vi "Test CML UI API.vi"() -> ()   [LabVIEW 2020]
doc: "CML UI API Tester.\n_____\nBased on DQMH Project Template 7.0.1.1316."
uses:
  <vilib>/Utility/error.llb/DialogType.ctl
  CML UI.lvlib
  <vilib>/Peloton/Peloton Config/DCFG Framework/Peloton_lib_DCFG Framework.lvlib
panel:
  in  "Views":string(combo)
  in  "Show DCFG Framework":bool
  in  "Show Diagram on Init":bool
  out "last error":errorcluster
  in  "Show Block Diagram":bool
  in  "Stop Module":bool
  in  "Start Module":bool
  in  "Hide Module Panel":bool
  in  "Show Module Panel":bool
  out "Status":string
  out "Module Running?":bool
  # "This VI tests the API for the Module."
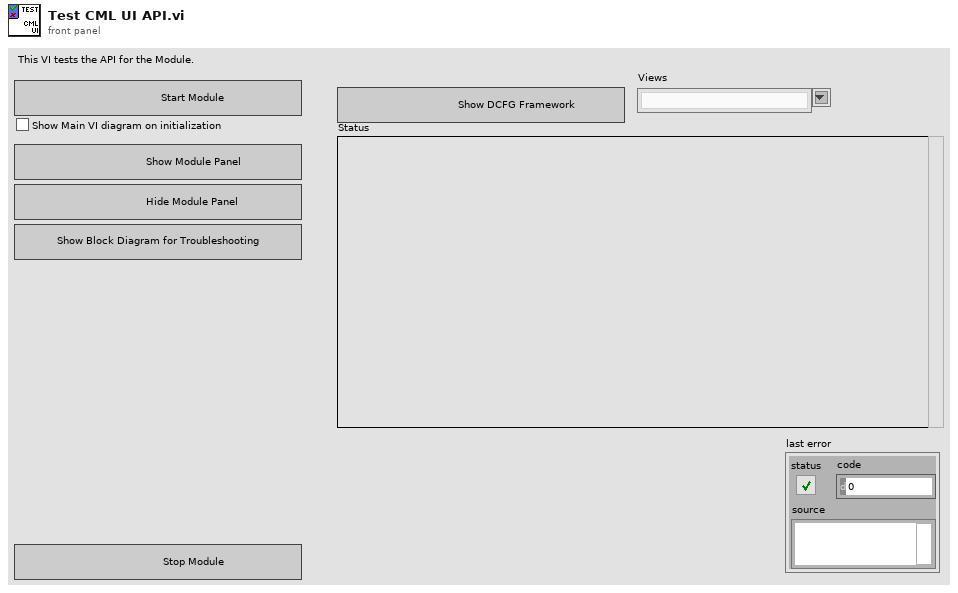
[diagram p1: front panel]
types:
  T1 = typedef "CML UI.lvlib/Broadcast Events--cluster.ctl" = cluster{"Module Did Init":refnum<user-event>, "Status Updated":refnum<user-event>, "Error Reported":refnum<user-event>, "Module Did Stop":refnum<user-event>, "Update Module Execution Status":refnum<user-event>}
  T2 = typedef "Peloton_lib_DCFG Framework.lvlib/Broadcast Events--cluster.ctl" = cluster{"Module Did Init":refnum<user-event>, "Status Updated":refnum<user-event>, "Error Reported":refnum<user-event>, "Module Did Stop":refnum<user-event>, "Update Module Execution Status":refnum<user-event>, "View Changed":refnum<user-event>, "Main Window Closed":refnum<user-event>, "Configuration Committed":refnum<user-event>, "Configuration Canceled":refnum<user-event>, "Views List Updated":refnum<user-event>, "Config Folder Path Updated":refnum<user-event>}
  T3 = typedef "DialogType.ctl" = u16
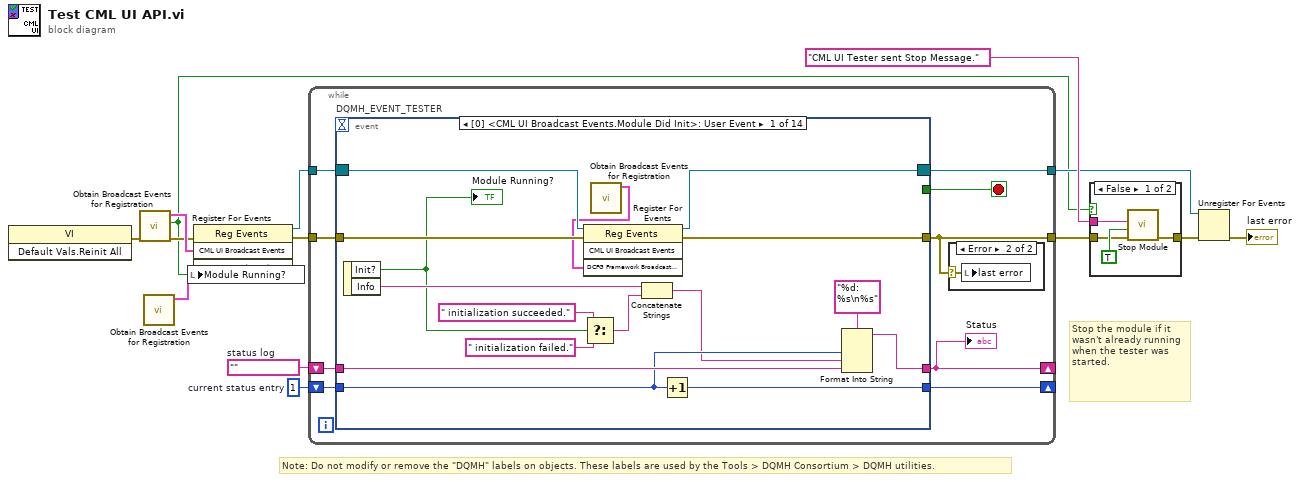
[diagram p0: block diagram]
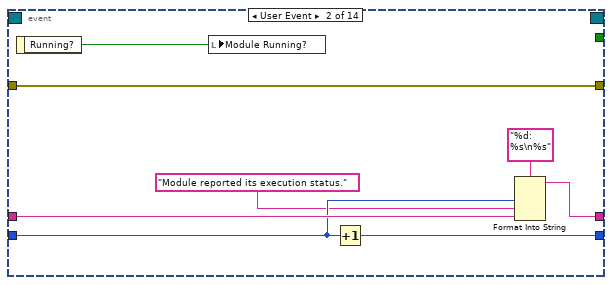
[diagram p3: hidden frame]
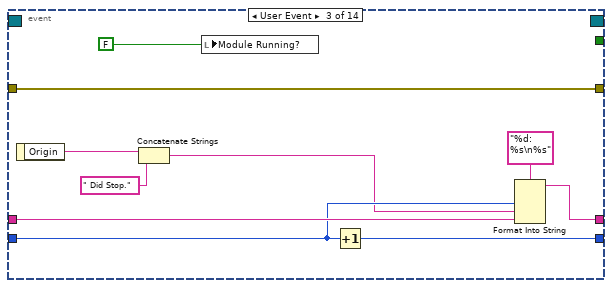
[diagram p4: hidden frame]
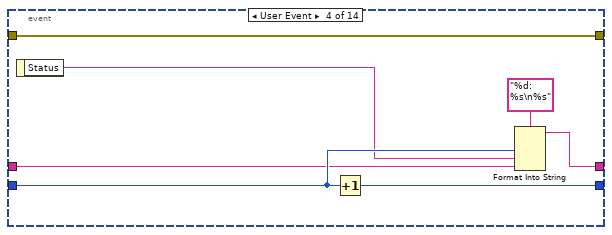
[diagram p5: hidden frame]
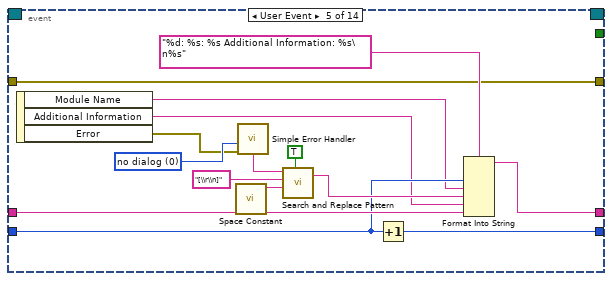
[diagram p6: hidden frame]
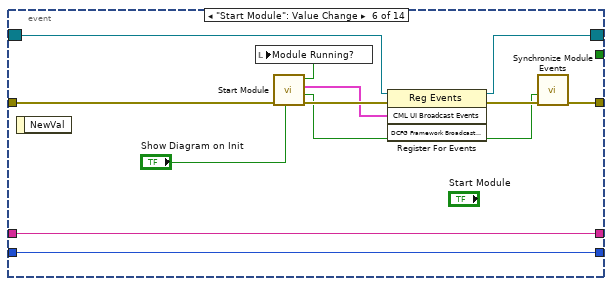
[diagram p7: hidden frame]
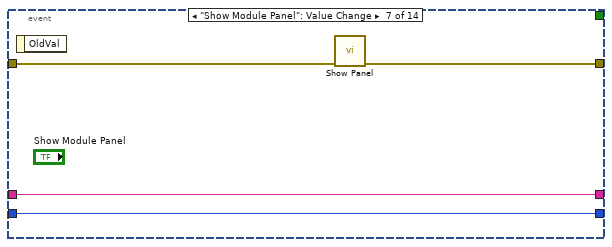
[diagram p8: hidden frame]
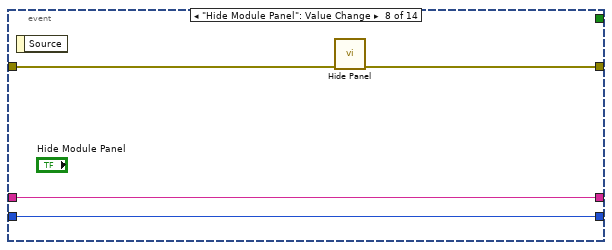
[diagram p9: hidden frame]
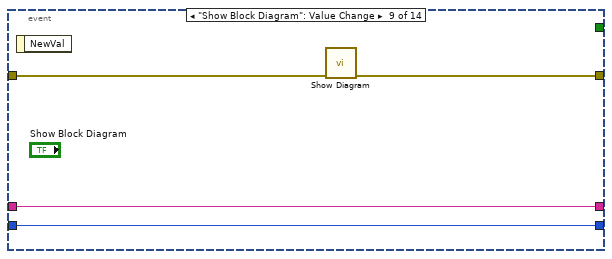
[diagram p10: hidden frame]
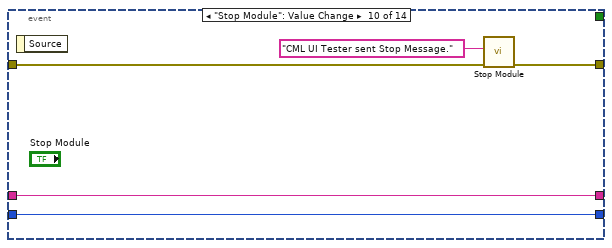
[diagram p11: hidden frame]
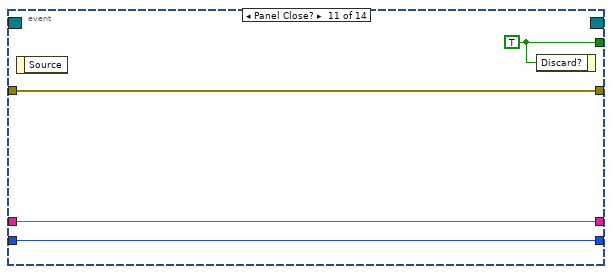
[diagram p12: hidden frame]
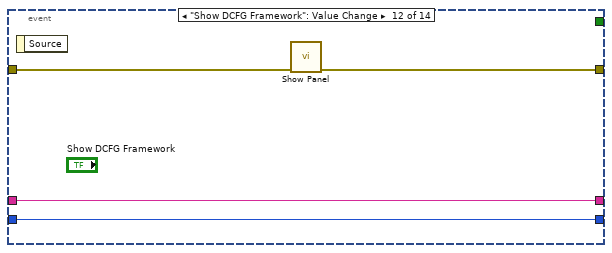
[diagram p13: hidden frame]
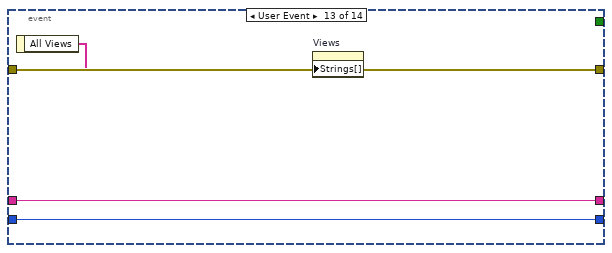
[diagram p14: hidden frame]
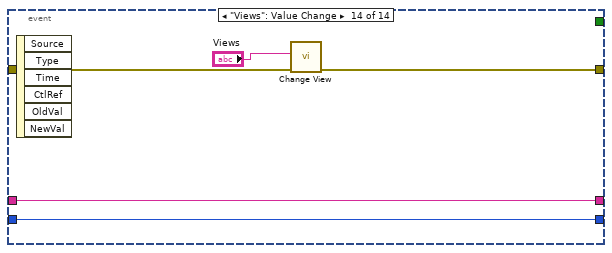
[diagram p15: hidden frame]
diagram:
  w11 = 1  # current status entry
  w12 = ""  # status log
  # "Stop the module if it wasn't already running when the tester was started."
  # "Note: Do not modify or remove the \"DQMH\" labels on objects. These labels are used by the Tools > DQMH Consortium > DQMH utilities."
  n1 = invoke class="VI" method="Default Vals.Reinit All"() -> (error out=w6:errorcluster)  [unwired: 3 in, 2 out]
  n2 = call <vilib>:"Obtain Broadcast Events for Registration.vi"("error in"=w6) -> ("error out"=w5:errorcluster, "Already running?"=w4:bool, "CML UI Broadcast Events"=w9:T1)  [unwired: 8 in]
  n3 = call <vilib>:"Obtain Broadcast Events for Registration.vi"() -> ("DCFG Framework Broadcast Events"=w1:T2)  [unwired: 9 in, 2 out]
  n4 = local write "Module Running?"(w4) -> ()
  n5 = register-events(error in=w5, w9, w1) -> (reference out=w8:refnum<event-registration>, error out=w10:errorcluster)  [unwired: 1 in]
  n6 = while {
    tunnel: w8 -> [w23]
    tunnel: [w15] -> w3
    shift-right: [w19] -> _
    shift-left: w12 -> [w21]
    shift-right: [w20] -> _
    shift-left: w11 -> [w22]
    tunnel: w10 -> [w18]
    tunnel: [w17] -> w7
    stop <- w16 stop-if-true
    n7 = event "DQMH_EVENT_TESTER" shown="[0] <CML UI Broadcast Events.Module Did Init>: User Event" {
      selector: w23 -> [w27 _ _ _ _ w86 _ _ _ _ _ _ _ _]
      dyn-events: [w26 _ _ _ _ w85 _ _ _ _ _ _ _ _] -> w17
      timeout: _ -> [_ _ _ _ _ _ _ _ _ _ _ _ _ _]
      tunnel: [_ _ _ _ _ _ _ _ _ _ w113 _ _ _] -> w16
      tunnel: [w28 w42 w49 w59 w69 w84 w96 w100 w101 w107 w110 w114 w121 w123] -> w15
      tunnel: w22 -> [w37 w46 w56 w62 w72 w89 w94 w98 w102 w108 w111 w115 w119 w124]
      tunnel: w21 -> [w38 w47 w57 w61 w73 w90 w95 w99 w103 w109 w112 w116 w120 w125]
      tunnel: [w35 w44 w54 w63 w71 w90 w95 w99 w103 w109 w112 w116 w120 w125] -> w19
      tunnel: [w36 w45 w55 w65 w70 w89 w94 w98 w102 w108 w111 w115 w119 w124] -> w20
      tunnel: w18 -> [w40 w42 w49 w59 w69 w83 w93 w97 w104 w105 w110 w117 w121 w126]
      event User Event {
        n8 = event-data() -> ("Init?"=w32:bool, "Info"=w34:string)  [unwired: 1 in]
        "Module Running?" <- w32
        n9 = Select(t=" initialization succeeded.", s=w32, f=" initialization failed.") -> (s? t:f=w29:string)
        n10 = call <vilib>:"Obtain Broadcast Events for Registration.vi"() -> ("DCFG Framework Broadcast Events"=w25:T2)  [unwired: 9 in, 2 out]
        n11 = register-events(reference=w27, error in=w40, w25) -> (reference out=w26:refnum<event-registration>, error out=w28:errorcluster)  [unwired: 1 in]
        n12 = Concatenate Strings(w34, w29) -> (w33:string)
        n13 = Increment(x=w37) -> (x+1=w36:i32)
        n14 = Format Into String(format string="%d: %s\n%s", w37, w33, w38) -> (resulting string=w35:string)  [unwired: 2 in, 1 out]
      }
      event User Event {
        n15 = event-data() -> ("Running?"=w41:bool)  [unwired: 1 in]
        n16 = local write "Module Running?"(w41) -> ()
        n17 = Increment(x=w46) -> (x+1=w45:i32)
        n18 = Format Into String(format string="%d: %s\n%s", w46, "Module reported its execution status.", w47) -> (resulting string=w44:string)  [unwired: 2 in, 1 out]
      }
      event User Event {
        n19 = event-data() -> ("Origin"=w53:string)  [unwired: 1 in]
        n20 = Concatenate Strings(w53, " Did Stop.") -> (w52:string)
        n21 = local write "Module Running?"(FALSE ("Module Did Init?")) -> ()
        n22 = Increment(x=w56) -> (x+1=w55:i32)
        n23 = Format Into String(format string="%d: %s\n%s", w56, w52, w57) -> (resulting string=w54:string)  [unwired: 2 in, 1 out]
      }
      event User Event {
        n24 = event-data() -> ("Status"=w60:string)  [unwired: 1 in]
        n25 = Increment(x=w62) -> (x+1=w65:i32)
        n26 = Format Into String(format string="%d: %s\n%s", w62, w60, w61) -> (resulting string=w63:string)  [unwired: 2 in, 1 out]
      }
      event User Event {
        w74 = T3 0 items=["no dialog", "OK message", "continue or stop message", "OK message + warnings", "continue/stop + warnings"] ("type of dialog (OK msg:1)")
        n27 = event-data() -> ("Module Name"=w68:string, "Additional Information"=w67:string, "Error"=w66:errorcluster)  [unwired: 1 in]
        n28 = call <vilib>:"Space Constant.vi"() -> ("String"=w78:string)
        n29 = call <vilib>:"Simple Error Handler.vi"("type of dialog (OK msg:1)"=w74, "error in (no error)"=w66) -> ("message"=w75:string)  [unwired: 3 in, 4 out]
        n30 = call <vilib>:"Search and Replace Pattern.vi"("string"=w75, "regular expression (\"\")"="[\\r\\n]" ("regular expression (\"\")"), "replace string (\"\")"=w78, "replace all? (F)"=TRUE ("replace all CR/LF with spaces")) -> ("result string"=w76:string)  [unwired: 1 in, 1 out]
        n31 = Increment(x=w72) -> (x+1=w70:i32)
        n32 = Format Into String(format string="%d: %s: %s Additional Information: %s\n%s", w72, w68, w76, w67, w73) -> (resulting string=w71:string)  [unwired: 2 in, 1 out]
      }
      event "Start Module": Value Change {
        n33 = event-data() -> ()  [unwired: 1 in, 1 out]
        n34 = call "Start Module.vi"("Show Main VI Diagram on Init (F)"="Show Diagram on Init", "error in"=w83) -> ("error out"=w91:errorcluster, "Wait for Event Sync?"=w88:bool, "CML UI Broadcast Events"=w87:T1, "Module Was Already Running?"=w82:bool)  [unwired: 6 in]
        n35 = local write "Module Running?"(w82) -> ()
        n36 = register-events(reference=w86, error in=w91, w87) -> (reference out=w85:refnum<event-registration>, error out=w92:errorcluster)  [unwired: 1 in]
        n37 = call "Synchronize Module Events.vi"("error in"=w92, "Wait for Event Sync?"=w88) -> ("error out"=w84:errorcluster)  [unwired: 9 in]
      }
      event "Show Module Panel": Value Change {
        n38 = event-data() -> ()  [unwired: 1 in, 1 out]
        n39 = call <vilib>:"Show Panel.vi"("error in"=w93) -> ("error out"=w96:errorcluster)  [unwired: 10 in]
      }
      event "Hide Module Panel": Value Change {
        n40 = event-data() -> ()  [unwired: 1 in, 1 out]
        n41 = call "Hide Panel.vi"("error in"=w97) -> ("error out"=w100:errorcluster)  [unwired: 10 in]
      }
      event "Show Block Diagram": Value Change {
        n42 = event-data() -> ()  [unwired: 1 in, 1 out]
        n43 = call "Show Diagram.vi"("error in"=w104) -> ("error out"=w101:errorcluster)  [unwired: 10 in]
      }
      event "Stop Module": Value Change {
        n44 = event-data() -> ()  [unwired: 1 in, 1 out]
        n45 = call "Stop Module.vi"("error in"=w105, "Origin"="CML UI Tester sent Stop Message.") -> ("error out"=w107:errorcluster)  [unwired: 9 in]
      }
      event Panel Close? {
        w113 = TRUE ("Discard?")
        n46 = event-data() -> ()  [unwired: 1 in, 1 out]
        n47 = event-data("Discard?"=w113) -> ()  [unwired: 1 in, 1 out]
      }
      event "Show DCFG Framework": Value Change {
        n48 = event-data() -> ()  [unwired: 1 in, 1 out]
        n49 = call <vilib>:"Show Panel.vi"("error in"=w117) -> ("error out"=w114:errorcluster)  [unwired: 10 in]
      }
      event User Event {
        n50 = event-data() -> ("All Views"=w118:string[])  [unwired: 1 in]
        n51 = property on="Views" class="CmbBox"("Strings[]"=w118) -> ()  [unwired: 2 in, 2 out]
      }
      event "Views": Value Change {
        n52 = event-data() -> ()  [unwired: 1 in, 6 out]
        n53 = call <vilib>:"Change View.vi"("error in"=w126, "View"="Views") -> ("error out"=w123:errorcluster)  [unwired: 9 in]
      }
    }
    "Status" <- w19
    n54 = case shown="Error" w15 {
      selector: w15 -> [_ w24]
      frame No Error {
      }
      frame Error {
        n55 = local write "last error"(w24) -> ()
      }
    }
  }
  n56 = case shown="False" w4 {
    tunnel: [w130 w131] -> w14
    tunnel: "CML UI Tester sent Stop Message." ("Origin") -> [w129 _]
    tunnel: w3 -> [w127 w131]
    frame False {
      n57 = call "Stop Module.vi"("error in"=w127, "Wait for Module to Stop? (F)"=TRUE ("Wait for Module to stop?"), "Origin"=w129) -> ("error out"=w130:errorcluster)  [unwired: 8 in]
    }
    frame True {
    }
  }
  n58 = Unregister For Events(event registration refnum=w7, error in=w14) -> (error out=→"last error":errorcluster)
